vi "pb_start.vi"(8 "error in (no error)":errorcluster, 11 "path in":path) -> (0 "error out":errorcluster, 3 "path out":path)   [LabVIEW 2016]
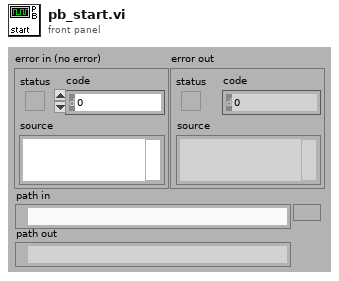
[diagram p1: front panel]
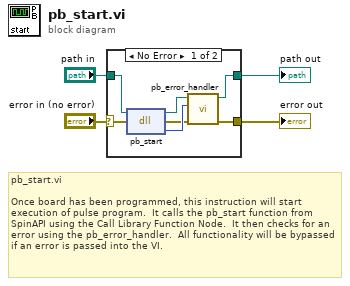
[diagram p0: block diagram]
diagram:
  # "pb_start.vi\n\nOnce board has been programmed, this instruction will start execution of pulse program.  It calls the pb_start function from SpinAPI using the Call Library Function Node.  It then checks for an error using the pb_error_handler.  All functionality will be bypassed if an error is passed into the VI."
  n1 = case shown="No Error" "error in (no error)" {
    selector: "error in (no error)" -> [w11 w13]
    tunnel: [w5 w13] -> w3
    tunnel: "path in" -> [w9 w12]
    tunnel: [w7 w12] -> w1
    frame No Error {
      n2 = dll-call lib="C:/Program Files/SpinCore/SpinAPI/dll/spinapi.dll" fn="pb_start"(path in=w9, error in=w11) -> (path out=w8:path, error out=w6:errorcluster, "return type"=w10:i32)  [unwired: 1 in]
      n3 = call "pb_error_handler.vi"("error in (no error)"=w6, "return code"=w10, "path in"=w8) -> ("error out"=w5:errorcluster, "path out"=w7:path)  [unwired: 7 out]
    }
    frame Error {
    }
  }
  "error out" <- w3
  "path out" <- w1
